vi "cvt_Enum_Init.vi"(8 "error in (no error)":errorcluster, 11 "Tag List":T1[](array[typedef])) -> (0 "error out":errorcluster)   [LabVIEW 2010]
uses:
  TypeDefs/cvt_TagList Methods.ctl
  TypeDefs/cvt_MemBlock Methods.ctl
  TypeDefs/cvt_Data Types.ctl
  TypeDefs/cvt_Tag Configuration.ctl
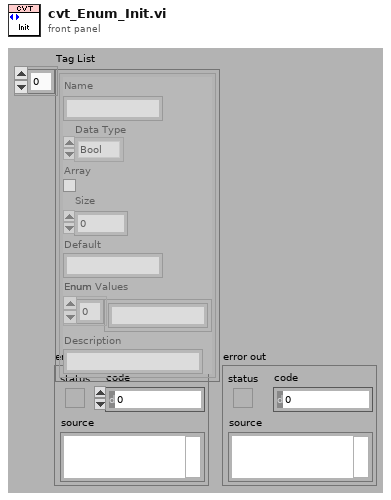
[diagram p1: front panel]
types:
  T1 = typedef "cvt_Tag Configuration.ctl" = cluster{"Name":string, "Data Type":T2, "Array":bool, "Size":u32, "Default":string, "Enum":string[], "Description":string}
  T2 = typedef "cvt_Data Types.ctl" = enum16{"Bool", "U8", "I32", "Double", "String", "Enum"}
  T3 = typedef "cvt_TagList Methods.ctl" = enum16{"init", "getindex", "getdesc", "getlist"}
  T4 = typedef "cvt_MemBlock Methods.ctl" = enum16{"init", "read", "readall", "write"}
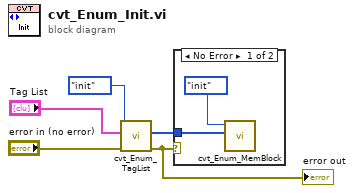
[diagram p0: block diagram]
diagram:
  n1 = call "cvt_Enum_TagList.vi"("error in (no error)"="error in (no error)", "Tag List"="Tag List", "Method"=cvt_TagList_Methods."init") -> ("error out"=w1:errorcluster, "Default Data"=w5:i32[])  [unwired: 1 in, 6 out]
  "error out" <- w1
  n2 = case shown="No Error" w1 {
    tunnel: w5 -> [w6 _]
    frame No Error {
      n3 = call "cvt_Enum_MemBlock.vi"("Default Data"=w6, "Method"=cvt_MemBlock_Methods."init") -> ()  [unwired: 2 in, 8 out]
    }
    frame Error {
    }
  }
